vi "IntakeNetwork.vi"(8 "error in (no error)":errorcluster) -> (0 "error out":errorcluster)   [LabVIEW 2020]
doc: "Intake Network\n\nInputs:\n -- Error in -- Error cluster -- propagated error input\n\nOutputs:\n -- Error out -- Error cluster -- progated error output"
uses:
  <vilib>/Rock Robotics/Network Tables/NT Write Number.vi
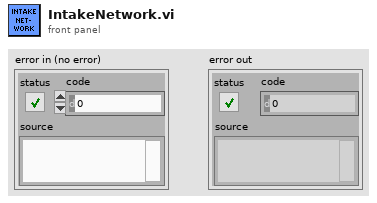
[diagram p1: front panel]
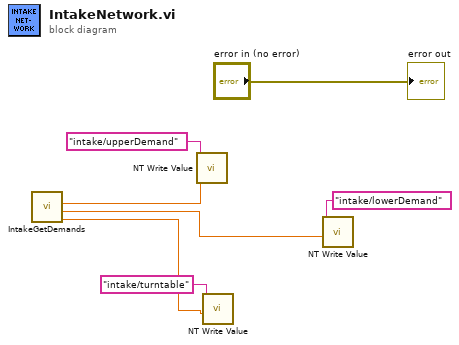
[diagram p0: block diagram]
diagram:
  n1 = call "IntakeGetDemands.vi"() -> ("turntableDemand"=w4:dbl, "intakeLowerDemand"=w5:dbl, "intakeUpperDemand"=w6:dbl)  [unwired: 9 in]
  n2 = call-poly <vilib>:"NT Write Value.vi"("value"=w6, "name"="intake/upperDemand") -> ()  [unwired: 9 in, 1 out]
  n3 = call-poly <vilib>:"NT Write Value.vi"("value"=w4, "name"="intake/turntable") -> ()  [unwired: 9 in, 1 out]
  n4 = call-poly <vilib>:"NT Write Value.vi"("value"=w5, "name"="intake/lowerDemand") -> ()  [unwired: 9 in, 1 out]
  "error out" <- "error in (no error)"
